vi "pthread_mutex_timedlock.vi"(8 "error in (no error)":errorcluster, 10 "absolute time":cluster{"sec":u64, "nsec":u64}, 11 "mutex ptr in":u64) -> (0 "error out":errorcluster, 2 "timed out?":bool, 3 "mutex ptr out":u64)   [LabVIEW 2016, in "Linux RT IPC.POSIX Threads.lvlib" / "POSIX Thread Object.lvclass"]
uses:
  POSIX Thread Object.lvclass
  Controls/pthread functions.ctl
  <vilib>/NI/NI Linux RT Errno/Controls/Public/errno.ctl
  <vilib>/NI/NI Linux RT Errno/Linux Errno.lvlib
  <vilib>/NI/NI Linux RT Utilities/Linux RT Utilities.lvlib
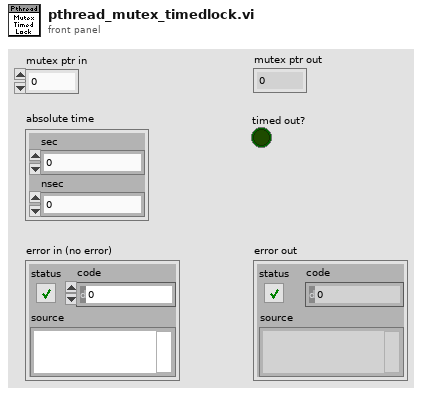
[diagram p1: front panel]
types:
  T1 = typedef "Linux Errno.lvlib/errno.ctl" = enum16{"NO ERROR", "EPERM", "ENOENT", "ESRCH", "EINTR", "EIO", "ENXIO", "E2BIG", "ENOEXEC", "EBADF", "ECHILD", "EAGAIN", "ENOMEM", "EACCES", "EFAULT", "ENOTBLK", "EBUSY", "EEXIST", "EXDEV", "ENODEV", "ENOTDIR", "EISDIR", "EINVAL", "ENFILE", "EMFILE", "ENOTTY", "ETXTBSY", "EFBIG", "ENOSPC", "ESPIPE", "EROFS", "EMLINK", "EPIPE", "EDOM", "ERANGE", "EDADLK", "ENAMETOOLONG", "ENOLCK", "ENOSYS", "ENOTEMPTY", "ELOOP", "EWOULDBLOCK", "ENOMSG", "EIDRM", "ECHRNG", "EL2NSYNC", "EL3HLT", "EL3RST", "ELNRNG", "EUNATCH", "ENOCSI", "EL2HLT", "EBADE", "EBADR", "EXFULL", "ENOANO", "EBADRQC", "EBADSLT", "EDEADLOCK", "EBFONT", "ENOSTR", "ENODATA", "ETIME", "ENOSR", "ENONET", "ENOPKG", "EREMOTE", "ENOLINK", "EADV", "ESRMNT", "ECOMM", "EPROTO", "EMULTIHOP", "EDOTDOT", "EBADMSG", "EOVERFLOW", "ENOTUNIQ", "EBADFD", "EREMCHG", "ELIBACC", "ELIBBAD", "ELIBSCN", "ELIBMAX", "ELIBEXEC", "ELISEQ", "ERESTART", "ESTRPIPE", "EUSERS", "ENOTSOCK", "EDESTADDRREQ", "EMSGSIZE", "EPROTOTYPE", "ENOPROTOOPT", "EPROTONOSUPPORT", "ESOCKTNOSUPPORT", "EOPNOTSUPP", "EPFNOSUPPORT", "EAFNOSUPPORT", "EADDRINUSE", "EADDRNOTAVAIL", "ENETDOWN", "ENETUNREACH", "ENETRESET", "ECONNABORTED", "ECONNRESET", "ENOBUFS", "EISCONN", "ENOTCONN", "ESHUTDOWN", "ETOOMANYREFS", "ETIMEDOUT", "ECONNREFUSED", "EHOSTDOWN", "EHOSTUNREACH", "EALREADY", "EINPROGRESS", "ESTALE", "EUCLEAN", "ENOTNAM", "ENAVAIL", "EISNAM", "EREMOTEIO", "EDQUOT", "ENOMEDIUM", "EMEDIUMTYPE", "ECANCELED", "ENOKEY", "EKEYEXPIRED", "EKEYREVOKED", "EKEYREJECTED", "EOWNERDEAD", "ENOTRECOVERABLE", "ERFKILL", "EHWPOISON", "UNDEFINED"}
  T2 = typedef "Linux RT IPC.POSIX Threads.lvlib/POSIX Thread Object.lvclass/pthread functions.ctl" = enum16{"unspecified", "pthread_condattr_init", "pthread_condattr_destroy", "pthread_condattr_getclock", "pthread_condattr_setclock", "pthread_condattr_getpshared", "pthread_condattr_setpshared", "pthread_cond_init", "pthread_cond_destroy", "pthread_cond_broadcast", "pthread_cond_signal", "pthread_cond_timedwait", "pthread_cond_wait", "pthread_mutexattr_init", "pthread_mutexattr_destroy", "pthread_mutexattr_getprioceiling", "pthread_mutexattr_setprioceiling", "pthread_mutexattr_getprotocol", "pthread_mutexattr_setprotocol", "pthread_mutexattr_getpshared", "pthread_mutexattr_setpshared", "pthread_mutexattr_gettype", "pthread_mutexattr_settype", "pthread_mutex_init", "pthread_mutex_destroy", "pthread_mutex_getprioceiling", "pthread_mutex_setprioceiling", "pthread_mutex_lock", "pthread_mutex_timedlock", "pthread_mutex_trylock", "pthread_mutex_unlock", "sem_destroy", "sem_getvalue", "sem_init", "sem_open", "sem_post", "sem_timedwait", "sem_trywait", "sem_wait", "barrier_init", "barrier_destroy", "barrier_wait", "barrierattr_init", "barrierattr_destroy", "barrierattr_getpshared", "barrierattr_setpshared"}
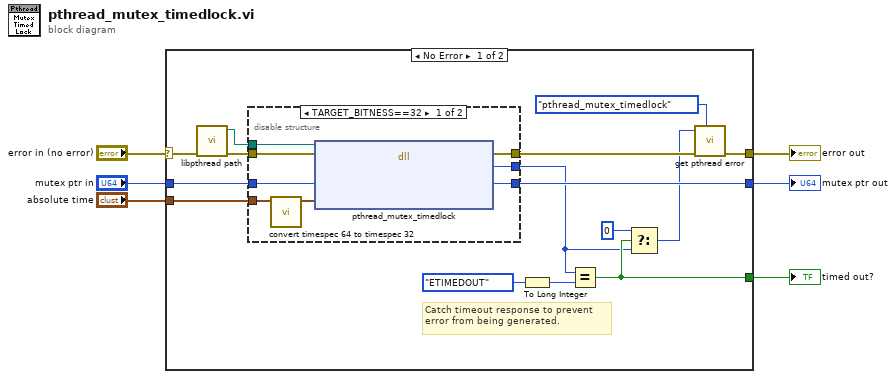
[diagram p0: block diagram]
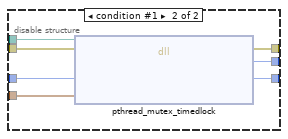
[diagram p2: hidden frame]
diagram:
  n1 = case shown="No Error" "error in (no error)" {
    selector: "error in (no error)" -> [w21 w38]
    tunnel: "mutex ptr in" -> [w9 w37]
    tunnel: [w20 w38] -> w4
    tunnel: [w12 w37] -> w3
    tunnel: "absolute time" -> [w7 _]
    tunnel: [w19 _] -> w1
    frame No Error {
      # "Catch timeout response to prevent error from being generated."
      n2 = call "libpthread path.vi"("error in (no error)"=w21) -> ("error out"=w14:errorcluster, "path to libpthread"=w8:path)  [unwired: 9 in]
      n3 = disable-structure shown="TARGET_BITNESS==32" {
        disable-tunnel: w14 -> [w29 w36]
        disable-tunnel: [w28 w35] -> w13
        disable-tunnel: [w27 w34] -> w12
        disable-tunnel: [w26 w33] -> w11
        disable-tunnel: w9 -> [w25 w32]
        disable-tunnel: w8 -> [w24 w31]
        disable-tunnel: w7 -> [w23 w30]
        frame condition #0 (active) {
          n4 = call <vilib>:"convert timespec 64 to timespec 32.vi"("timespec 64"=w23) -> ("timespec 32"=w22:cluster{"sec":u32, "nsec":u32})  [unwired: 10 in]
          n5 = dll-call lib="?" fn="pthread_mutex_timedlock"(path in=w24, error in=w29, "mutex"=w25, "abstime"=w22) -> (error out=w28:errorcluster, "errno"=w26:i32, "mutex"=w27:u64)  [unwired: 2 in, 1 out]
        }
        frame condition #1 {
          n6 = dll-call lib="?" fn="pthread_mutex_timedlock"(path in=w31, error in=w36, "mutex"=w32, "abstime"=w30) -> (error out=w35:errorcluster, "errno"=w33:i32, "mutex"=w34:u64)  [unwired: 2 in, 1 out]
        }
      }
      n7 = To Long Integer(number=errno."ETIMEDOUT" ("errno")) -> (32bit integer=w17:i32)
      n8 = Equal?(x=w11, y=w17) -> (x = y?=w19:bool)
      n9 = Select(t=0, s=w19, f=w11) -> (s? t:f=w10:i32)
      n10 = call "get pthread error.vi"("function"=pthread_functions."pthread_mutex_timedlock", "error in (no error)"=w13, "errno"=w10) -> ("error out"=w20:errorcluster)  [unwired: 8 in]
    }
    frame Error {
    }
  }
  "error out" <- w4
  "mutex ptr out" <- w3
  "timed out?" <- w1
